vi "Obtain Doc Title.vi"(8 "error in (no error)":errorcluster, 11 "Py Editor in":refnum<class "Py Editor.lvclass">) -> (0 "error out":errorcluster, 3 "Py Editor out":refnum<class "Py Editor.lvclass">)   [LabVIEW 2019, in "Py Editor.lvclass"]
uses:
  Py Editor.lvclass
  D:/Namratha/MDI/LabVIEW-MDI-develop_LV2019/source code/Document/Py Doc/Py Doc.lvclass
  D:/Namratha/MDI/LabVIEW-MDI-develop_LV2019/source code/Document/Document base/Document.lvclass
  Py Doc.lvclass/Py Doc.ctl
  Document base/Document.lvclass/Document.ctl
  Property/Read Py File Path.vi
  Document base/property/Write Doc Title.vi
  <vilib>/regexp/Match Regular Expression.xnode
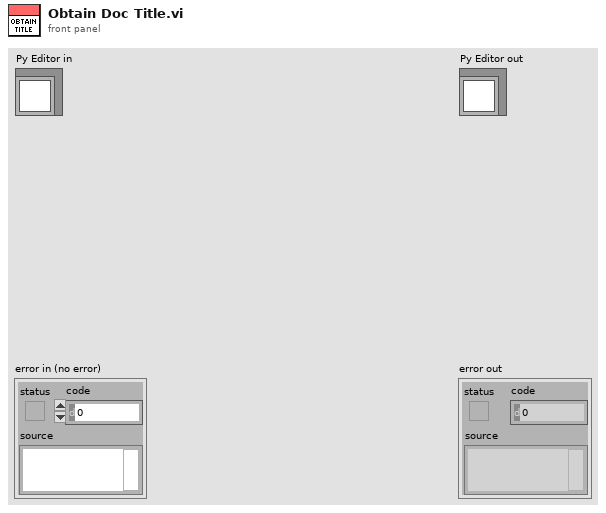
[diagram p1: front panel]
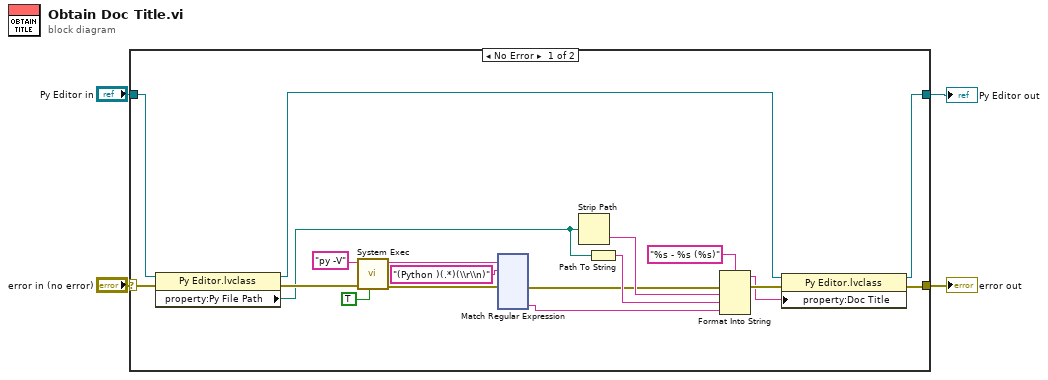
[diagram p0: block diagram]
diagram:
  n1 = case shown="No Error" "error in (no error)" {
    selector: "error in (no error)" -> [w12 w141]
    tunnel: [w8 w141] -> w3
    tunnel: "Py Editor in" -> [w9 w142]
    tunnel: [w6 w142] -> w1
    frame No Error {
      n2 = property class="Py Editor.lvclass"(reference=w9, error in=w12) -> (reference out=w7:refnum<class "Py Editor.lvclass">, error out=w11:errorcluster, "property:Py File Path"=w10:path)
      n3 = call <vilib>:"System Exec.vi"("run minimized? (F)"=TRUE, "error in (no error)"=w11, "command line"="py -V") -> ("error out"=w14:errorcluster, "standard output"=w15:string)  [unwired: 5 in, 2 out]
      n4 = xnode "Match Regular Expression"("input string"=w15, "regular expression"="(Python )(.*)(\\r\\n)", "error in"=w14) -> ("error out"=w19:errorcluster, "submatch 2"=w18:string)  [unwired: 3 in, 5 out]
      n5 = Strip Path(path=w10) -> (name=w21:string)  [unwired: 1 out]
      n6 = Path To String(path=w10) -> (string=w23:string)
      n7 = Format Into String(format string="%s - %s (%s)", error in=w19, w21, w23, w18) -> (resulting string=w5:string, error out=w20:errorcluster)  [unwired: 1 in]
      n8 = property class="Py Editor.lvclass"(reference=w7, error in=w20, "property:Doc Title"=w5) -> (reference out=w6:refnum<class "Py Editor.lvclass">, error out=w8:errorcluster)
    }
    frame Error {
    }
  }
  "error out" <- w3
  "Py Editor out" <- w1
